vi "geve-msg_macro_kill_application.vi"(10 "Kill log message":string, 11 "Runtime Data in":T1) -> ()   [LabVIEW 2018]
doc: "enqueue actions to worker :\n\nlog stop message, and send stop request."
uses:
  geve-runtime_data_cluster.ctl
  geve-monitoring_data_cluster.ctl
  geve-serial_config_cluster.ctl
  geve-com_ref_cluster.ctl
  geve-message_cluster.ctl
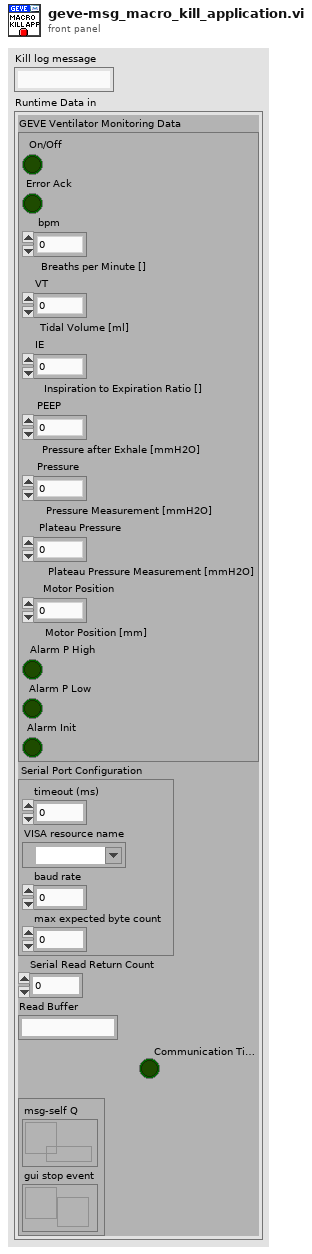
[diagram p1: front panel]
types:
  T1 = typedef "geve-runtime_data_cluster.ctl" = cluster{"GEVE Ventilator Monitoring Data":T2, "Serial Port Configuration":T3, "Serial Read Return Count":u32, "Read Buffer":string, "Communication Timeout?":bool, "com-refs":T4}
  T2 = typedef "geve-monitoring_data_cluster.ctl" = cluster{"On/Off":bool, "Error Ack":bool, "bpm":dbl, "VT":dbl, "IE":dbl, "PEEP":dbl, "Pressure":dbl, "Plateau Pressure":dbl, "Motor Position":dbl, "Alarm P High":bool, "Alarm P Low":bool, "Alarm Init":bool}
  T3 = typedef "geve-serial_config_cluster.ctl" = cluster{"timeout (ms)":u32, "VISA resource name":refnum<visa-resource-name>, "baud rate":u32, "max expected byte count":u32}
  T4 = typedef "geve-com_ref_cluster.ctl" = cluster{"msg-self Q":refnum<queue>, "gui stop event":refnum<user-event>}
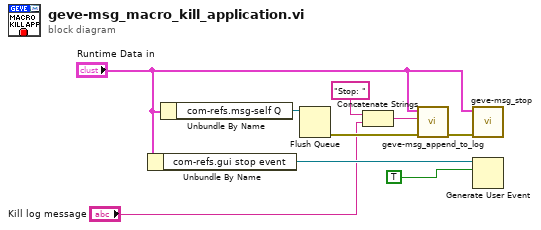
[diagram p0: block diagram]
diagram:
  n1 = Unbundle By Name("Runtime Data in") -> ("com-refs.gui stop event"=w8:refnum<user-event>)
  n2 = Unbundle By Name("Runtime Data in") -> ("com-refs.msg-self Q"=w6:refnum<queue>)
  n3 = Flush Queue(queue=w6) -> (error out=w5:errorcluster)  [unwired: 1 in, 2 out]
  n4 = Concatenate Strings("Stop: " ("Status Message"), "Kill log message") -> (w3:string)
  n5 = call "geve-msg_append_to_log.vi"("error in (no error)"=w5, "Status Message"=w3, "Runtime Data"="Runtime Data in") -> ("error out"=w4:errorcluster)  [unwired: 7 in, 1 out]
  n6 = call "geve-msg_stop.vi"("error in (no error)"=w4, "Runtime Data"="Runtime Data in") -> ()  [unwired: 8 in, 2 out]
  n7 = Generate User Event(user event=w8, event data cluster=TRUE ("event data")) -> ()  [unwired: 2 in, 2 out]
